vi "rotate_about_axis.vi"(8 "Angle":dbl, 9 "Axis":cluster{"X":dbl, "Y":dbl, "Z":dbl}={"X"=0.0, "Y"=1.0, "Z"=0.0}, 10 "Vector":cluster{"X":dbl, "Y":dbl, "Z":dbl}={"X"=0.0, "Y"=1.0, "Z"=0.0}) -> (2 "Rotated Vector":T1)   [LabVIEW 2020, in "3DPC_SurfacePlot.xctl"]
uses:
  <vilib>/Native 3D Graph/xcontrol/3DPC_SurfacePlot.xctl
  <vilib>/Analysis/baseanly.llb/A x Vector.vi
  <vilib>/Analysis/NI_AALBase.lvlib
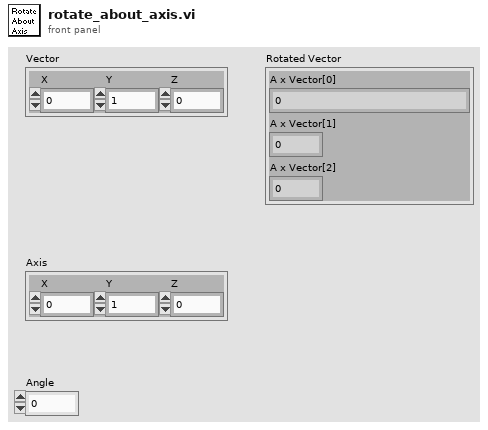
[diagram p1: front panel]
types:
  T1 = cluster{"A x Vector[0]":dbl, "A x Vector[1]":dbl, "A x Vector[2]":dbl}
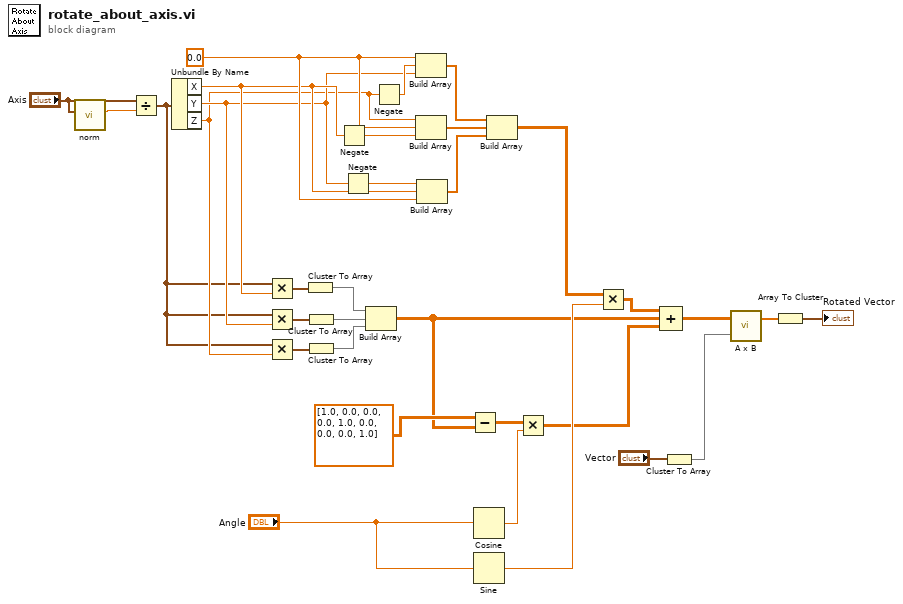
[diagram p0: block diagram]
diagram:
  w29 = 0.0 ("Angle")
  n1 = call <vilib>:"norm.vi"("Vector"="Axis") -> ("Norm"=w1:sgl)  [unwired: 10 out]
  n2 = Divide(x="Axis", y=w1) -> (x/y=w22:cluster{"X":dbl, "Y":dbl, "Z":dbl})
  n3 = Unbundle By Name(w22) -> ("X"=w25:dbl, "Y"=w24:dbl, "Z"=w23:dbl)
  n4 = Multiply(x=w22, y=w25) -> (x*y=w21:cluster{"X":dbl, "Y":dbl, "Z":dbl})
  n5 = Multiply(x=w22, y=w24) -> (x*y=w20:cluster{"X":dbl, "Y":dbl, "Z":dbl})
  n6 = Multiply(x=w22, y=w23) -> (x*y=w19:cluster{"X":dbl, "Y":dbl, "Z":dbl})
  n7 = Cluster To Array(cluster=w21) -> (array=w18:dbl[])
  n8 = Cluster To Array(cluster=w20) -> (array=w17:dbl[])
  n9 = Cluster To Array(cluster=w19) -> (array=w16:dbl[])
  n10 = Negate(x=w25) -> (-x=w32:dbl)
  n11 = Negate(x=w24) -> (-x=w30:dbl)
  n12 = Build Array(w18, w17, w16) -> (w8:dbl[][])
  n13 = Negate(x=w23) -> (-x=w31:dbl)
  n14 = Build Array(w29, w31, w24) -> (w28:dbl[])
  n15 = Build Array(w23, w29, w32) -> (w27:dbl[])
  n16 = Build Array(w30, w25, w29) -> (w26:dbl[])
  n17 = Subtract(x=dbl[][] [[1.0, 0.0, 0.0], [0.0, 1.0, 0.0], [0.0, 0.0, 1.0]] ("appended array"), y=w8) -> (x-y=w13:dbl[][])
  n18 = Cosine(x="Angle") -> (cos(x)=w14:dbl)
  n19 = Sine(x="Angle") -> (sin(x)=w10:dbl)
  n20 = Build Array(w28, w27, w26) -> (w11:dbl[][])
  n21 = Multiply(x=w13, y=w14) -> (x*y=w7:dbl[][])
  n22 = Multiply(x=w11, y=w10) -> (x*y=w9:dbl[][])
  n23 = Compound Arithmetic op=ADD(w9, w8, w7) -> (w5:dbl[][])
  n24 = Cluster To Array(cluster="Vector") -> (array=w4:dbl[])
  n25 = call-poly <vilib>:"A x B.vi"("Vector"=w4, "A"=w5) -> ("A x Vector"=w3:dbl[])  [unwired: 1 out]
  n26 = Array To Cluster(array=w3) -> (cluster=→"Rotated Vector":T1)
